vi "SENS_CORR_COLL_GUID_ADAP_CRE.vi"(0 "VISA IN":refnum<visa-resource-name>, 1 "Port 1 Conn Type":string, 2 "Port 2 Conn Type":string, 5 "error in":errorcluster, 7 "Channel":i32) -> (14 "VISA Out":refnum<visa-resource-name>, 16 "Data":dbl, 19 "error out":errorcluster)   [LabVIEW 2018, in "PNA-X.lvlib"]
doc: "SENSe<cnum>:CORRection:COLLect:GUIDed:ADAPter:CREate? <conn1>, <conn2> \n(Read-only) Specifies the use of a THRU adapter to be used during the Guided Cal Unknown THRU \nand Adapter Removal Cal. Returns an adapter index <n> which is used to refer to the adapter in \nseveral related commands. See Cal Thru Methods. While the choice of which end of the adapter is \n<conn1> and <conn2> is arbitrary, it is necessary to remember which will be used on each test port. \nParameters \n<cnum> Any existing channel number. If unspecified, value is set to 1 \n<conn1> Adapter port 1 connector type. Use SENS:CORR:COLL:GUID:CONN:CAT? \nto return a list of valid connector types. \n<conn2> Adapter port 2 connector type. \nExamples See example using this command. \nReturn Type Numeric \n1643\n\nDefault Not Applicable"
uses:
  PNA-X.lvlib
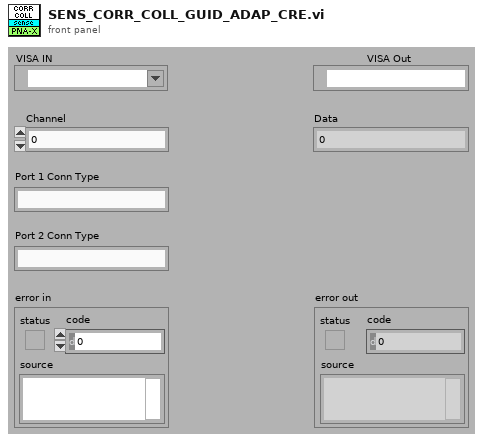
[diagram p1: front panel]
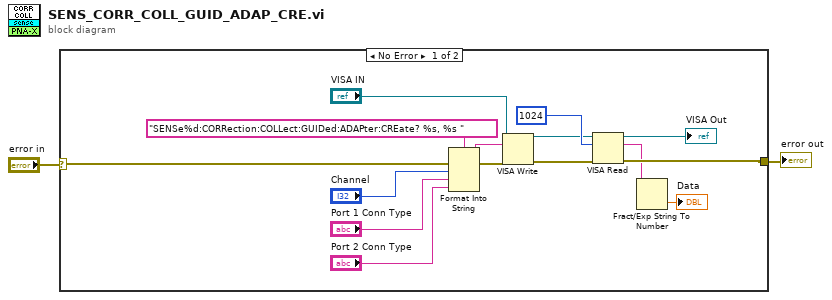
[diagram p0: block diagram]
diagram:
  n1 = case shown="No Error" "error in" {
    selector: "error in" -> [w17 w18]
    tunnel: [w8 w18] -> w1
    frame No Error {
      n2 = Format Into String(format string="SENSe%d:CORRection:COLLect:GUIDed:ADAPter:CREate? %s, %s " ("Cmdline"), error in=w17, "Channel", "Port 1 Conn Type", "Port 2 Conn Type") -> (resulting string=w15:string, error out=w16:errorcluster)  [unwired: 1 in]
      n3 = VISA Write(VISA resource name="VISA IN", write buffer=w15, error in (no error)=w16) -> (VISA resource name out=w10:refnum<visa-resource-name>, error out=w12:errorcluster)  [unwired: 1 out]
      n4 = VISA Read(VISA resource name=w10, byte count=1024, error in (no error)=w12) -> (VISA resource name out=→"VISA Out":refnum<visa-resource-name>, read buffer=w6:string, error out=w8:errorcluster)  [unwired: 1 out]
      n5 = Fract/Exp String To Number(string=w6) -> (number=→"Data":dbl)  [unwired: 3 in, 1 out]
    }
    frame Error {
    }
  }
  "error out" <- w1
